vi "Sonar - Max&Kevin.vi"() -> (3 "distance":dbl(slide)=125.0 scale=0.0..250.0 scale format="%3d", 4 "error out":errorcluster)   [LabVIEW 2012]
doc: "This example shows how to use the MaxBotix LV-MaxSonar-EZ1 Sonar Range Finder MB1010. It will display the distance from the sensor in inches.\n\nThis example works with the NI 9403 module connected to a Digital Sidecar. The Digital Sidecar should have 12V applied to the WAGO connector. The sensor is attached to the 3x8 header using a 3-pin PWM connector."
uses:
  <vilib>/Rock Robotics/SystemInterfaces/DIO/FPGA_DIOChannel.ctl
  <vilib>/Rock Robotics/SystemInterfaces/Typedef/FPGA_TypedefDigitalModule.ctl
  <vilib>/Rock Robotics/WPI/Counter/WPI_CounterDigitalInputToDigitalSource.vi
  <vilib>/Rock Robotics/WPI/Counter/WPI_CounterOpen Semi Period Mode.vi
panel:
  out "M2 output":dbl
  in  "M2 input":dbl
  out "M1 Output":dbl
  in  "M1 input":dbl
  out "error out 2":errorcluster
  out "distance 2":dbl(slide)=125.0 scale=0.0..250.0 scale format="%3d"
  # "Output information."
  # "EZ1"
  # "inches"
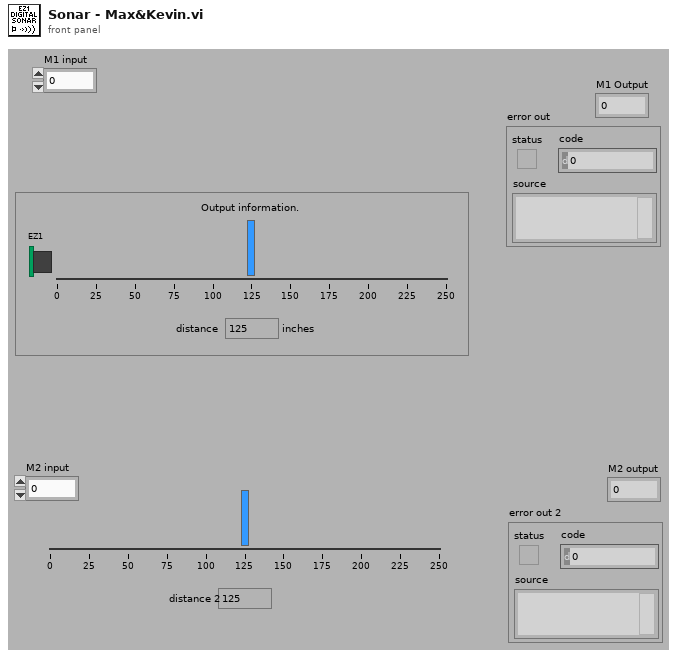
[diagram p1: front panel]
types:
  T1 = typedef "FPGA_DIOChannel.ctl" = enum8{"DIO 1", "DIO 2", "DIO 3", "DIO 4", "DIO 5", "DIO 6", "DIO 7", "DIO 8", "DIO 9", "DIO 10", "DIO 11", "DIO 12", "DIO 13", "DIO 14", "Invalid"}
  T2 = typedef "FPGA_TypedefDigitalModule.ctl" = enum16{"Digital Module 1", "Digital Module 2"}
  T3 = typedef "WPI_DigitalInputDevRef.ctl" = cluster{"DevStatus":errorcluster, "DIO Channel":T1, "Digital Module":T2}
  T4 = typedef "FPGA_CounterEncoderSourceConvertionLVSourceType.ctl" = cluster{"DevStatus":errorcluster, "AnalogTriggerMode?":bool, "DigitalMode":cluster{"Digital Module":T2, "DIO Channel":T5}, "AnalogTriggerMode":cluster{"AnalogTriggerIndex":T6, "OutputType":T7}}
  T5 = typedef "FPGA_DIODigitalSourceChannel.ctl" = enum8{"DIO 1", "DIO 2", "DIO 3", "DIO 4", "DIO 5", "DIO 6", "DIO 7", "DIO 8", "DIO 9", "DIO 10", "DIO 11", "DIO 12", "DIO 13", "DIO 14", "Disabled"}
  T6 = typedef "FPGA_AnalogTriggerIndex.ctl" = enum8{"Trig 0", "Trig 1", "Trig 2", "Trig 3", "Trig 4", "Trig 5", "Trig 6", "Trig 7", "Invalid"}
  T7 = typedef "FPGA_AnalogTriggerOutType.ctl" = enum16{"InWindow", "TriggerState", "Rising", "Falling"}
  T8 = typedef "WPI_CounterDevRef.ctl" = cluster{"DevStatus":errorcluster, "CntIndex":T9}
  T9 = typedef "FPGA_CounterCtrSystemIndex.ctl" = enum8{"Ctr 0", "Ctr 1", "Ctr 2", "Ctr 3", "Ctr 4", "Ctr 5", "Ctr 6", "Ctr 7", "Invalid"}
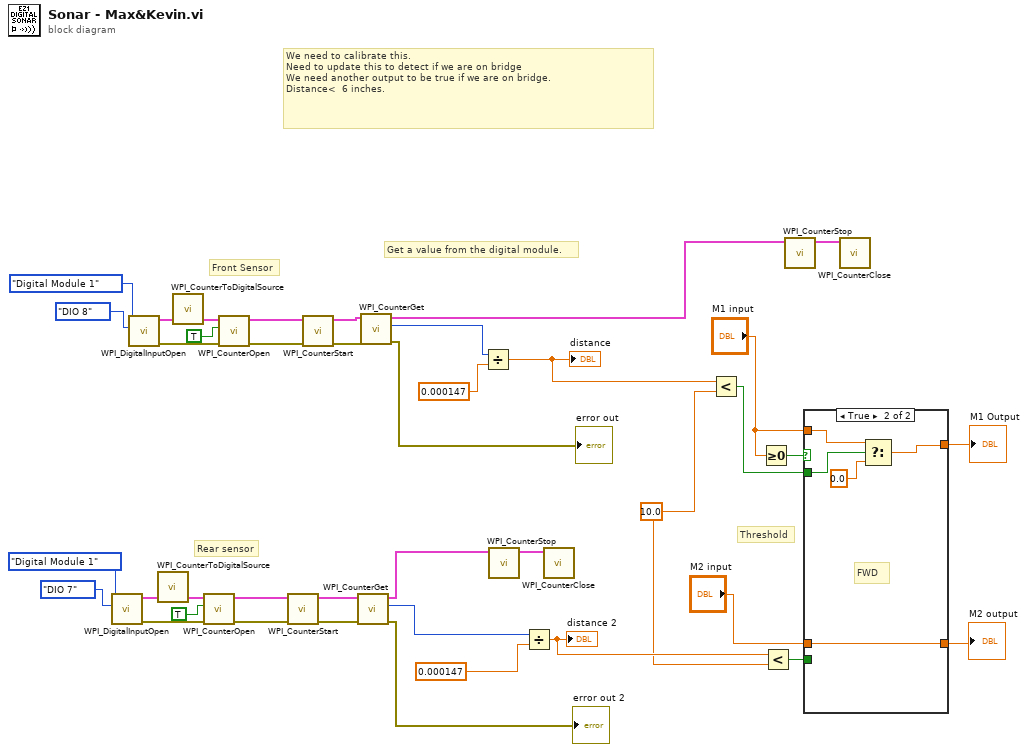
[diagram p0: block diagram]
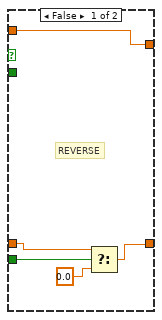
[diagram p2: hidden frame]
diagram:
  w32 = 10.0 ("y")
  # "Rear sensor"
  # "Front Sensor"
  # "Threshold"
  # "We need to calibrate this.\nNeed to update this to detect if we are on bridge\nWe need another output to be true if we are on bridge.\nDistance<  6 inches."
  # "Get a value from the digital module."
  n1 = call <vilib>:"WPI_DigitalInputOpen.vi"("DIO Channel"=FPGA_DIOChannel."DIO 7", "Digital Module (Module 1)"=FPGA_TypedefDigitalModule."Digital Module 1" ("DIO Module")) -> ("error out"=w13:errorcluster, "DigitalInputDevRef"=w2:T3)  [unwired: 1 in, 7 out]
  n2 = call <vilib>:"WPI_DigitalInputOpen.vi"("DIO Channel"=FPGA_DIOChannel."DIO 8", "Digital Module (Module 1)"=FPGA_TypedefDigitalModule."Digital Module 1" ("DIO Module")) -> ("error out"=w16:errorcluster, "DigitalInputDevRef"=w28:T3)  [unwired: 1 in, 7 out]
  n3 = call-poly <vilib>:"WPI_CounterToDigitalSource.vi"("DigitalInputDevRef"=w2) -> ("Digital Source"=w23:T4)  [unwired: 6 in]
  n4 = call-poly <vilib>:"WPI_CounterToDigitalSource.vi"("DigitalInputDevRef"=w28) -> ("Digital Source"=w30:T4)  [unwired: 6 in]
  n5 = call-poly <vilib>:"WPI_CounterOpen.vi"("error in (no error)"=w13, "High Pulse (T)"=TRUE, "Source"=w23) -> ("error out"=w12:errorcluster, "CounterDevRef"=w22:T8)  [unwired: 7 in]
  n6 = call-poly <vilib>:"WPI_CounterOpen.vi"("error in (no error)"=w16, "High Pulse (T)"=TRUE, "Source"=w30) -> ("error out"=w15:errorcluster, "CounterDevRef"=w29:T8)  [unwired: 7 in]
  n7 = call <vilib>:"WPI_CounterStart.vi"("error in (no error)"=w12, "CounterDevRef in"=w22) -> ("error out"=w11:errorcluster, "CounterDevRef out"=w20:T8)  [unwired: 8 in]
  n8 = call <vilib>:"WPI_CounterStart.vi"("error in (no error)"=w15, "CounterDevRef in"=w29) -> ("error out"=w14:errorcluster, "CounterDevRef out"=w26:T8)  [unwired: 8 in]
  n9 = call <vilib>:"WPI_CounterGet.vi"("error in (no error)"=w11, "CounterDevRef in"=w20) -> ("error out"=→"error out 2":errorcluster, "Value"=w35:i32, "CounterDevRef out"=w17:T8)  [unwired: 4 in, 3 out]
  n10 = call <vilib>:"WPI_CounterGet.vi"("error in (no error)"=w14, "CounterDevRef in"=w26) -> ("error out"=→"error out":errorcluster, "Value"=w38:i32, "CounterDevRef out"=w10:T8)  [unwired: 4 in, 3 out]
  n11 = Divide(x=w38, y=0.000147 ("Scaling factor (s/in)")) -> (x/y=w34:dbl)
  "distance" <- w34
  n12 = call <vilib>:"WPI_CounterStop.vi"("CounterDevRef in"=w17) -> ("CounterDevRef out"=w19:T8)  [unwired: 9 in, 1 out]
  n13 = Divide(x=w35, y=0.000147 ("Scaling factor (s/in)")) -> (x/y=w33:dbl)
  "distance 2" <- w33
  n14 = call <vilib>:"WPI_CounterClose.vi"("CounterDevRef"=w19) -> ()  [unwired: 10 in, 1 out]
  n15 = Less?(x=w34, y=w32) -> (x < y?=w6:bool)
  n16 = Greater Or Equal To 0?(x="M1 input") -> (x >= 0?=w9:bool)
  n17 = Less?(x=w33, y=w32) -> (x < y?=w3:bool)
  n18 = call <vilib>:"WPI_CounterStop.vi"("CounterDevRef in"=w10) -> ("CounterDevRef out"=w25:T8)  [unwired: 9 in, 1 out]
  n19 = case shown="True" w9 {
    tunnel: "M1 input" -> [w45 w47]
    tunnel: [w45 w49] -> w7
    tunnel: w6 -> [_ w48]
    tunnel: "M2 input" -> [w43 w46]
    tunnel: [w42 w46] -> w4
    tunnel: w3 -> [w41 _]
    frame False {
      # "REVERSE"
      n20 = Select(t=w43, s=w41, f=0.0) -> (s? t:f=w42:dbl)
    }
    frame True {
      # "FWD"
      n21 = Select(t=w47, s=w48, f=0.0) -> (s? t:f=w49:dbl)
    }
  }
  "M1 Output" <- w7
  "M2 output" <- w4
  n22 = call <vilib>:"WPI_CounterClose.vi"("CounterDevRef"=w25) -> ()  [unwired: 10 in, 1 out]
